vi "UnDecorator.vi"(8 "error in (no error)":errorcluster, 11 "DataVer2 in":refnum<class "DataVer2.lvclass">) -> (0 "error out":errorcluster, 2 "DecoratorData Out":refnum<class "Data.lvclass">, 3 "DataVer2 out":refnum<class "DataVer2.lvclass">)   [LabVIEW 2013, in "DataVer2.lvclass"]
uses:
  DataVer2.lvclass
  Data.lvclass/Data.lvclass
  DataVer2.lvclass/DataVer2.ctl
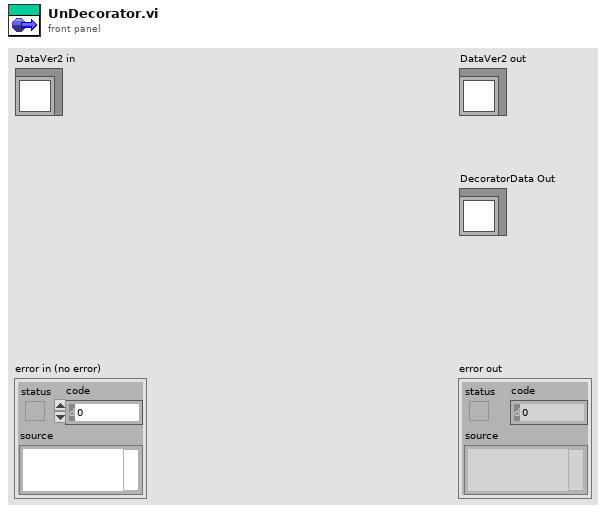
[diagram p1: front panel]
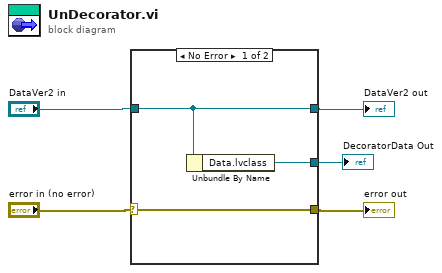
[diagram p0: block diagram]
diagram:
  n1 = case shown="No Error" "error in (no error)" {
    selector: "error in (no error)" -> [w8 w10]
    tunnel: [w8 w10] -> w5
    tunnel: [w7 w9] -> w4
    tunnel: "DataVer2 in" -> [w7 w9]
    tunnel: [w6 _] -> w1
    frame No Error {
      n2 = Unbundle By Name(w7) -> ("Data.lvclass"=w6:refnum<class "Data.lvclass">)
    }
    frame Error {
    }
  }
  "error out" <- w5
  "DataVer2 out" <- w4
  "DecoratorData Out" <- w1
